vi "Charact Path.vi"(0 "Path in":refnum<class "Path.lvclass">, 5 "Standard Type":T1, 11 "error in":errorcluster) -> (4 "Path out":refnum<class "Path.lvclass">, 6 "Aborted":bool, 15 "error out":errorcluster)   [LabVIEW 2023, in "RFFixtureCharact.Public.lvlib"]
uses:
  RFFixtureCharact.Public.lvlib
  Common/Base Classes/Path/Path.lvclass
  Instruments/Cal Standard/Type Definitions/Standard Type.ctl
  Instruments/RFFixtureCharact.Instruments.lvlib
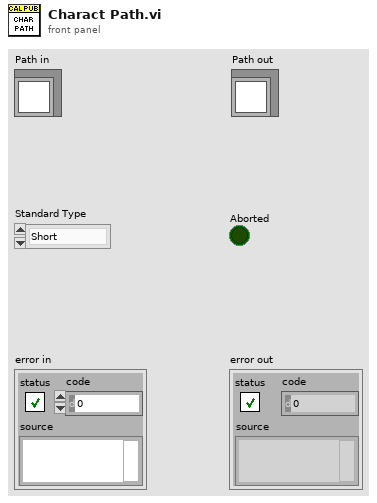
[diagram p1: front panel]
types:
  T1 = typedef "RFFixtureCharact.Instruments.lvlib/Standard Type.ctl" = enum16{"Short", "Open", "Load", "PowerMeter", "None"}
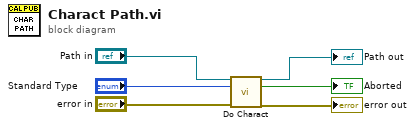
[diagram p0: block diagram]
diagram:
  n1 = call-dynamic "Do Charact.vi"("Path in"="Path in", "Charact Standard"="Standard Type", "error in (no error)"="error in") -> ("Path out"=→"Path out":refnum<class "Path.lvclass">, "Aborted"=→"Aborted":bool, "error out"=→"error out":errorcluster)  [unwired: 10 in]
